vi "plot_xy.vi"(5 "arrays in":cluster{dbl[], dbl[]}, 9 "selected":bool, 11 "XY Graph ref in":refnum<vi>) -> (3 "XY Graph ref out":refnum<vi>)   [LabVIEW 2015]
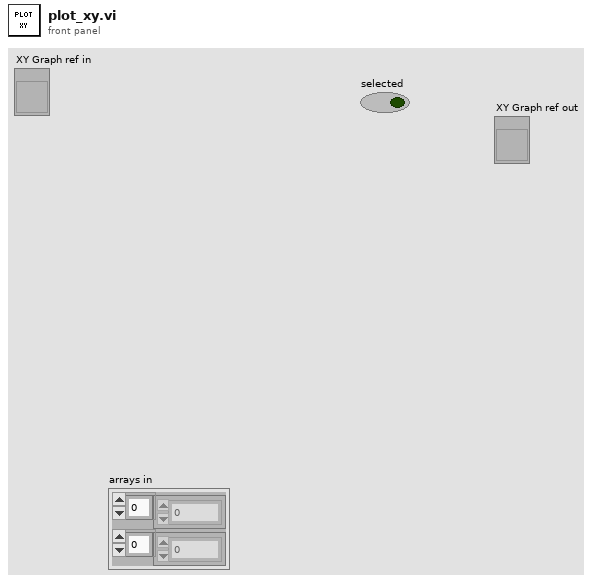
[diagram p1: front panel]
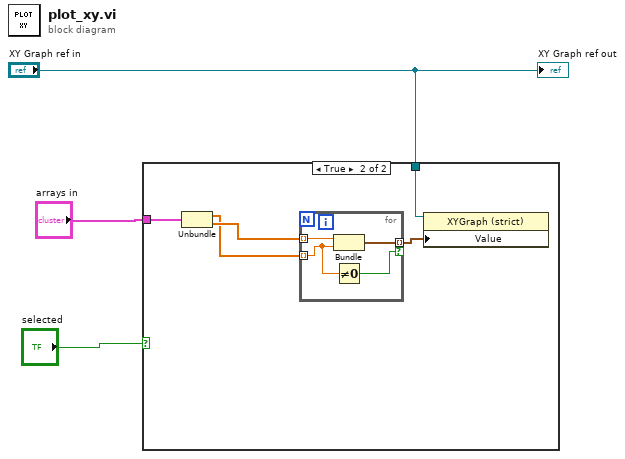
[diagram p0: block diagram]
diagram:
  n1 = case shown="True" "selected" {
    tunnel: "XY Graph ref in" -> [_ w8]
    tunnel: "arrays in" -> [_ w7]
    frame False {
    }
    frame True {
      n2 = Unbundle(w7) -> (w5:dbl[], w6:dbl[])
      n3 = for {
        tunnel: w6 -> [w12] mode=indexing
        tunnel: w5 -> [w10] mode=indexing
        tunnel: [w11] -> w4 mode=indexing if=w9
        n4 = Bundle("element"=w12, "element"=w10) -> (w11:cluster{"element":dbl, "element":dbl})  [unwired: 1 in]
        n5 = Not Equal To 0?(x=w10) -> (x != 0?=w9:bool)
      }
      n6 = property on="Property Node" class="XYGraph (strict)"(reference=w8, "Value"=w4) -> ()  [unwired: 1 in, 2 out]
    }
  }
  "XY Graph ref out" <- "XY Graph ref in"
